vi "Error Query.vi"(8 "error in (no error)":errorcluster, 11 "VISA resource name":refnum<visa-resource-name>) -> (0 "error out":errorcluster, 1 "Error Message":string, 2 "Error Code":i32[](array[numeric]), 3 "VISA resource name out":refnum<visa-resource-name>)   [LabVIEW 2020, in "Agilent 3446X Series.lvlib"]
doc: "Queries the instrument for any errors in the instrument's error queue. It will continue to read errors until all errors have been read from the instrument. Any errors will be returned in the <B>error out</B> control.\n\n<B>Note:</B>\nThis VI is called automatically by most driver VIs so it is not usually necessary to call this in an application."
uses:
  Agilent 3446X Series.lvlib
  681f8946-a6b3-4e84-9bae-842e8ea990b9.vi
  b8627da9-8d60-4db4-8425-39ea97d70fc7.vi
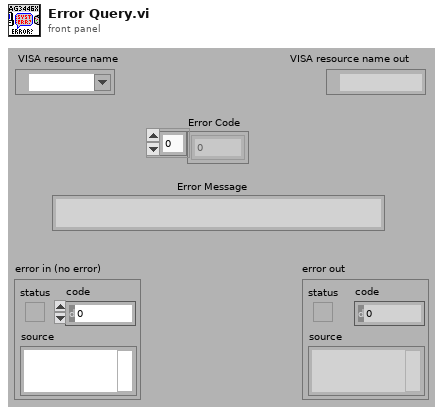
[diagram p1: front panel]
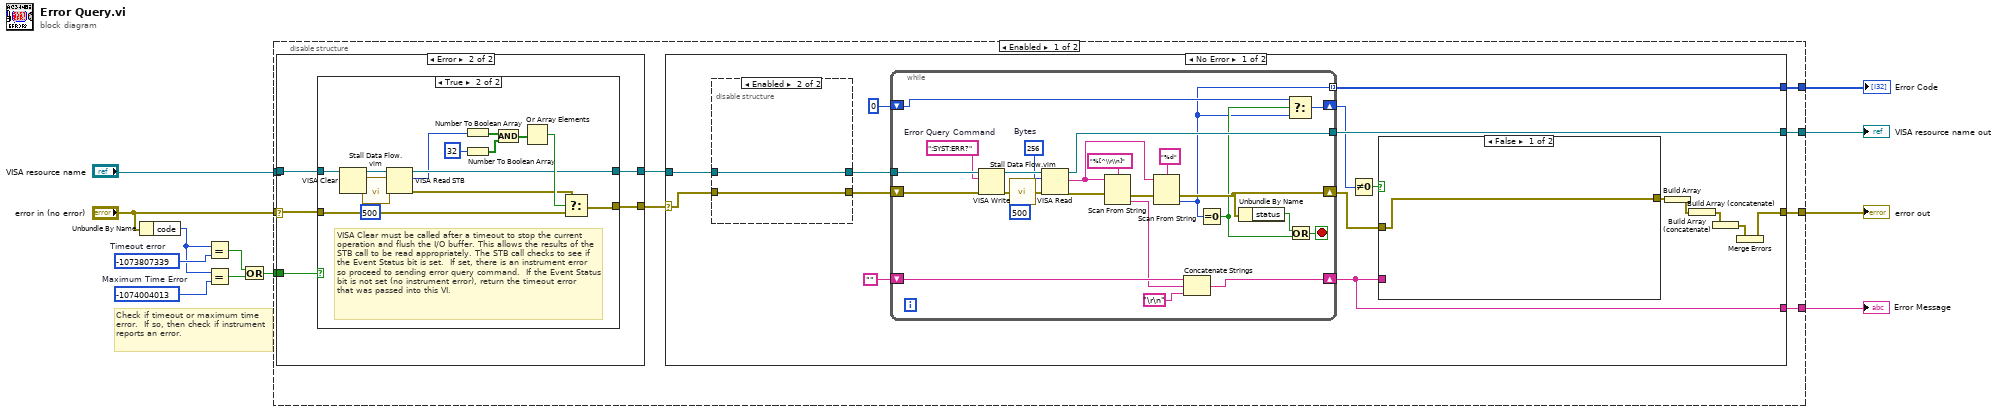
[diagram p0: block diagram]
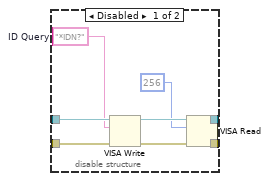
[diagram p4: hidden frame]
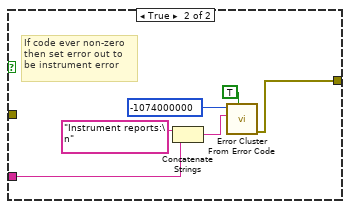
[diagram p5: hidden frame]
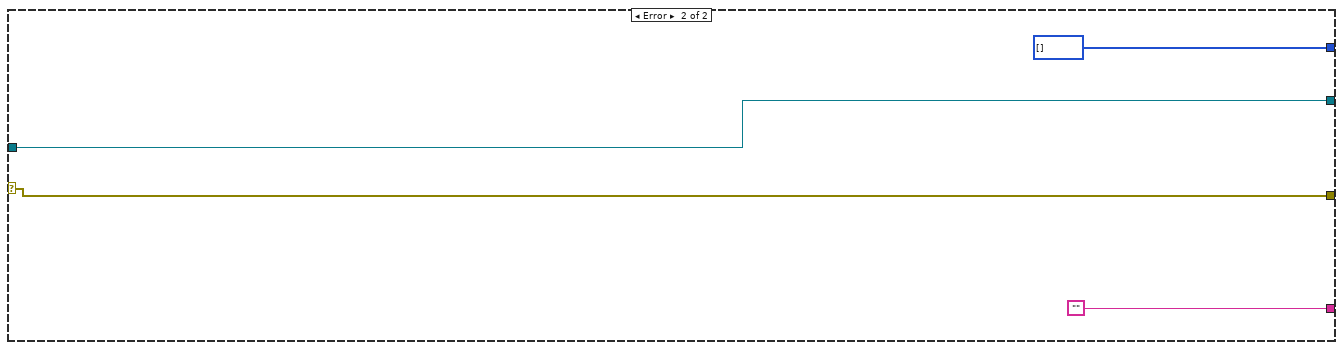
[diagram p6: hidden frame]
diagram:
  w5 = -1074004013  # Maximum Time Error
  w7 = -1073807339  # Timeout error
  # "Check if timeout or maximum time error.  If so, then check if instrument reports an error."
  n1 = Unbundle By Name("error in (no error)") -> ("code"=w6:i32)
  n2 = Equal?(x=w6, y=w7) -> (x = y?=w3:bool)
  n3 = Equal?(x=w6, y=w5) -> (x = y?=w4:bool)
  n4 = Or(x=w3, y=w4) -> (x .or. y?=w2:bool)
  n5 = disable-structure shown="Enabled" {
    disable-tunnel: [w21 w110] -> w12
    disable-tunnel: [w20 w109] -> w11
    disable-tunnel: [w19 _] -> w10
    disable-tunnel: [w18 _] -> w9
    disable-tunnel: "VISA resource name" -> [w15 w110]
    disable-tunnel: w2 -> [w14 _]
    disable-tunnel: "error in (no error)" -> [w13 w109]
    frame Enabled {
      n6 = case shown="Error" w13 {
        selector: w13 -> [w22 w26]
        tunnel: w15 -> [w23 w28]
        tunnel: [w23 w27] -> w16
        tunnel: [w22 w25] -> w17
        tunnel: w14 -> [_ w24]
        frame No Error {
        }
        frame Error {
          n7 = case shown="True" w24 {
            tunnel: w28 -> [w30 w38]
            tunnel: [w30 w35] -> w27
            tunnel: w26 -> [w29 w41]
            tunnel: [w29 w40] -> w25
            frame False {
              # "Error code not a timeout, so best to pass on to user."
            }
            frame True {
              # "VISA Clear must be called after a timeout to stop the current operation and flush the I/O buffer. This allows the results of the  STB call to be read appropriately. The STB call checks to see if the Event Status bit is set.  If set, there is an instrument error so proceed to sending error query command.  If the Event Status bit is not set (no instrument error), return the timeout error that was passed into this VI."
              n8 = VISA Clear(VISA resource name=w38) -> (VISA resource name out=w37:refnum<visa-resource-name>, error out=w36:errorcluster)  [unwired: 1 in]
              n9 = call "Stall Data Flow.vim"("value in"=w36, "milliseconds to wait"=u32 500) -> ("value out"=w32:errorcluster)  [unwired: 1 out]
              n10 = VISA Read STB(8:w32, 11:w37) -> (0:w34:errorcluster, 2:w33:u16, 3:w35:refnum<visa-resource-name>)
              n11 = Number To Boolean Array(number=w33) -> (Boolean array=w42:bool[])
              n12 = Number To Boolean Array(number=32) -> (Boolean array=w44:bool[])
              n13 = And(x=w42, y=w44) -> (x .and. y?=w43:bool[])
              n14 = Or Array Elements(Boolean array=w43) -> (logical OR=w39:bool)
              n15 = Select(t=w34, s=w39, f=w41) -> (s? t:f=w40:errorcluster)
            }
          }
        }
      }
      n16 = case shown="No Error" w17 {
        selector: w17 -> [w52 w105]
        tunnel: [w62 w108] -> w21
        tunnel: w16 -> [w48 w108]
        tunnel: [w60 w105] -> w20
        tunnel: [w55 ""] -> w19
        tunnel: [w54 i32[] []] -> w18
        frame No Error {
          n17 = disable-structure shown="Enabled" {
            disable-tunnel: w52 -> [w70 w71]
            disable-tunnel: w48 -> [w68 w72]
            disable-tunnel: [w67 w71] -> w47
            disable-tunnel: [w65 w72] -> w46
            frame Disabled {
              w63 = "*IDN?"  # ID Query
              n18 = VISA Write(VISA resource name=w68, write buffer=w63, error in (no error)=w70) -> (VISA resource name out=w66:refnum<visa-resource-name>, error out=w69:errorcluster)  [unwired: 1 out]
              n19 = VISA Read(VISA resource name=w66, byte count=u32 256, error in (no error)=w69) -> (VISA resource name out=w65:refnum<visa-resource-name>, error out=w67:errorcluster)  [unwired: 2 out]
            }
            frame Enabled {
            }
          }
          n20 = while {
            tunnel: [w104] -> w62
            tunnel: w46 -> [w103]
            shift-right: [w91] -> w55
            shift-left: "" -> [w94]
            shift-right: [w89] -> w56
            shift-left: 0 -> [w90]
            shift-right: [w87] -> w53
            shift-left: w47 -> [w88]
            tunnel: [w82] -> w54 mode=indexing
            stop <- w97 stop-if-true
            w101 = u32 256  # Bytes
            w99 = ":SYST:ERR?"  # Error Query Command
            n21 = VISA Write(VISA resource name=w103, write buffer=w99, error in (no error)=w88) -> (VISA resource name out=w102:refnum<visa-resource-name>, error out=w100:errorcluster)  [unwired: 1 out]
            n22 = call "Stall Data Flow.vim"("value in"=w100, "milliseconds to wait"=u32 500) -> ("value out"=w81:errorcluster)  [unwired: 1 out]
            n23 = VISA Read(VISA resource name=w102, byte count=w101, error in (no error)=w81) -> (VISA resource name out=w104:refnum<visa-resource-name>, read buffer=w95:string, error out=w86:errorcluster)  [unwired: 1 out]
            n24 = Scan From String(format string="%[^\\r\\n]", input string=w95, error in=w86) -> (error out=w85:errorcluster, output 1=w92:string)  [unwired: 1 in, 3 out]
            n25 = Scan From String(format string="%d", input string=w95, error in=w85) -> (error out=w87:errorcluster, output 1=w82:i32)  [unwired: 1 in, 3 out]
            n26 = Concatenate Strings(w94, w92, "\r\n") -> (w91:string)
            n27 = Equal To 0?(x=w82) -> (x = 0?=w83:bool)
            n28 = Unbundle By Name(w87) -> ("status"=w84:bool)
            n29 = Select(t=w90, s=w83, f=w82) -> (s? t:f=w89:i32)
            n30 = Or(x=w84, y=w83) -> (x .or. y?=w97:bool)
          }
          n31 = Not Equal To 0?(x=w56) -> (x != 0?=w58:bool)
          n32 = case shown="False" w58 {
            tunnel: w55 -> [_ w78]
            tunnel: [w73 w74] -> w57
            tunnel: w53 -> [w73 _]
            frame False {
            }
            frame True {
              # "If code ever non-zero\nthen set error out to\nbe instrument error"
              n33 = Concatenate Strings("Instrument reports:\n" ("Source"), w78) -> (w75:string)
              n34 = call <vilib>:"Error Cluster From Error Code.vi"("show call chain? (False)"=TRUE, "error message (\"\")"=w75, "error code (0)"=-1074000000 ("Code")) -> ("error out"=w74:errorcluster)  [unwired: 1 in, 5 out]
            }
          }
          n35 = Build Array(w57) -> (w51:errorcluster[])
          n36 = Build Array (concatenate)(w51) -> (w50:errorcluster[])
          n37 = Build Array (concatenate)(w50) -> (w49:errorcluster[])
          n38 = Merge Errors(w49) -> (w60:errorcluster)
        }
        frame Error {
        }
      }
    }
    frame Disabled {
    }
  }
  "VISA resource name out" <- w12
  "error out" <- w11
  "Error Message" <- w10
  "Error Code" <- w9
